vi "Read File to Parse.vi"(8 "error in (no error)":errorcluster, 11 "File Parsing Interface in":refnum<class "File Parsing Interface.lvclass">) -> (0 "error out":errorcluster, 2 "File to Parse":path, 3 "File Parsing Interface out":refnum<class "File Parsing Interface.lvclass">)   [LabVIEW 2018, in "File Parsing Interface.lvlib" / "File Parsing Interface.lvclass"]
uses:
  File Parsing Interface.lvclass
  File Parsing Interface.lvclass/File Parsing Interface.ctl
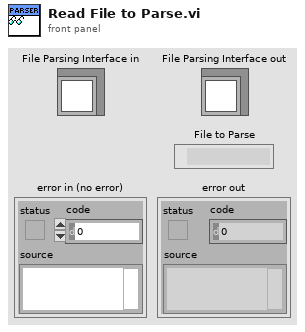
[diagram p1: front panel]
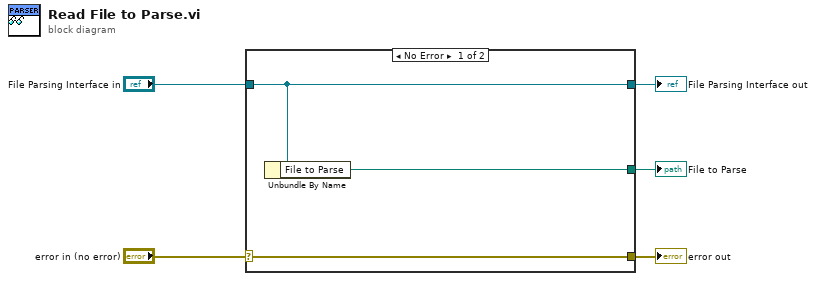
[diagram p0: block diagram]
diagram:
  n1 = case shown="No Error" "error in (no error)" {
    selector: "error in (no error)" -> [w8 w9]
    tunnel: [w8 w9] -> w4
    tunnel: [w7 w10] -> w2
    tunnel: "File Parsing Interface in" -> [w7 w10]
    tunnel: [w6 _] -> w1
    frame No Error {
      n2 = Unbundle By Name(w7) -> ("File to Parse"=w6:path)
    }
    frame Error {
    }
  }
  "error out" <- w4
  "File Parsing Interface out" <- w2
  "File to Parse" <- w1
